vi "timeUnit.set.vi"(8 "error in (no error)":errorcluster, 10 "timeUnit":T1(ring), 11 "ts.epochOfTimeUnit in":refnum<class "ts.epochOfTimeUnit.lvclass">) -> (0 "error out":errorcluster, 3 "ts.epochOfTimeUnit out":refnum<class "ts.epochOfTimeUnit.lvclass">)   [LabVIEW 2020, in "ts.epochOfTimeUnit.lvclass"]
uses:
  ts.epochOfTimeUnit.lvclass
  ts.epochOfTimeUnit.lvclass/ts.epochOfTimeUnit.ctl
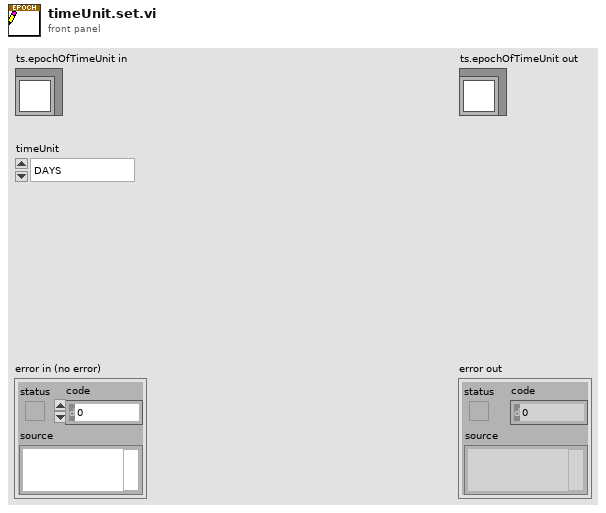
[diagram p1: front panel]
types:
  T1 = enum16{"DAYS", "HOURS", "MINUTES", "SECONDS", "MILLISECONDS", "MICROSECONDS", "NANOSECONDS", "PICOSECONDS"}
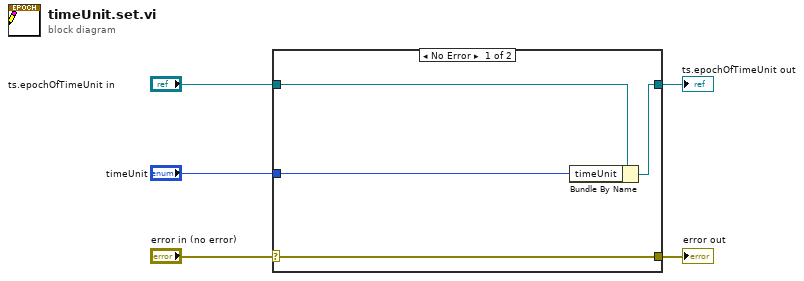
[diagram p0: block diagram]
diagram:
  n1 = case shown="No Error" "error in (no error)" {
    selector: "error in (no error)" -> [w9 w10]
    tunnel: [w9 w10] -> w4
    tunnel: [w7 w11] -> w2
    tunnel: "ts.epochOfTimeUnit in" -> [w8 w11]
    tunnel: "timeUnit" -> [w6 _]
    frame No Error {
      n2 = Bundle By Name(cluster=w8, "timeUnit"=w6) -> (w7:refnum<class "ts.epochOfTimeUnit.lvclass">)
    }
    frame Error {
    }
  }
  "error out" <- w4
  "ts.epochOfTimeUnit out" <- w2
